vi "Get Device Reference.vi"(11 "CD_Process in":refnum<class "Process.lvclass">) -> (2 "Device Item Ref":T1=18446744073709551615 format="%.0x", 3 "CD_Process out":refnum<class "Process.lvclass">)   [LabVIEW 2019, in "TimingDRV Engine.lvlib" / "Process.lvclass"]
uses:
  Process.lvclass
  <vilib>/NI VeriStand/Custom Device API/Custom Device Item Ref.ctl
  Process.lvclass/Process.ctl
  <vilib>/NI VeriStand/Custom Device API/Custom Device API.lvlib
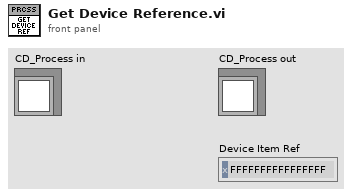
[diagram p1: front panel]
types:
  T1 = typedef "Custom Device API.lvlib/Custom Device Item Ref.ctl" = u64
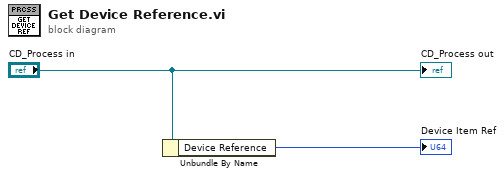
[diagram p0: block diagram]
diagram:
  n1 = Unbundle By Name("CD_Process in") -> ("Device Reference"=→"Device Item Ref":T1)
  "CD_Process out" <- "CD_Process in"
